vi "SelectCurDigital2DListCtrl.vi"(7 "clicked seq list?":bool, 8 "digital":dbl, 9 "digital in":refnum<vi>, 10 "column index":u16, 11 "list in":refnum<vi>) -> (3 "list out":refnum<vi>)   [LabVIEW 2018, in "Library-Ctrl.lvlib"]
uses:
  Library-Ctrl.lvlib
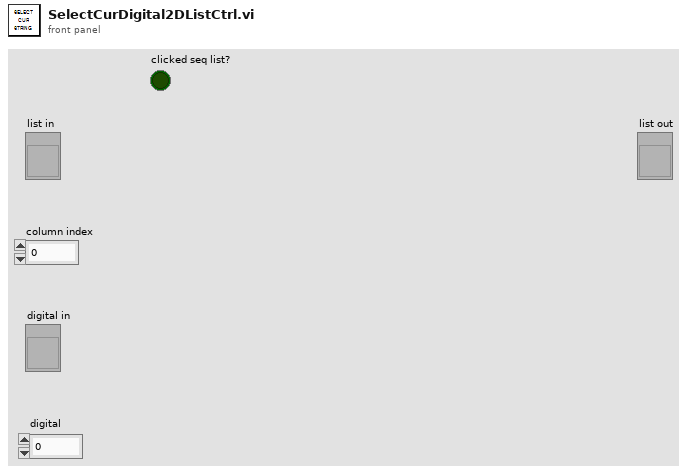
[diagram p1: front panel]
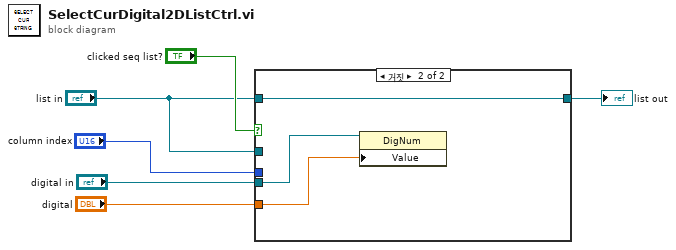
[diagram p0: block diagram]
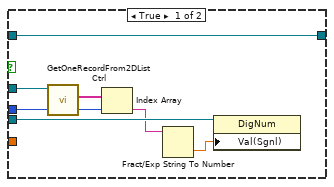
[diagram p2: hidden frame]
diagram:
  n1 = case shown="거짓" "clicked seq list?" {
    tunnel: "digital in" -> [w11 w16]
    tunnel: "digital" -> [_ w15]
    tunnel: "list in" -> [w13 _]
    tunnel: "column index" -> [w10 _]
    tunnel: [w9 w14] -> w2
    tunnel: "list in" -> [w9 w14]
    frame True {
      n2 = call "GetOneRecordFrom2DListCtrl.vi"("testcaselist in"=w13) -> ("one record"=w12:string[])  [unwired: 9 in, 1 out]
      n3 = Index Array(array=w12, index=w10) -> (element=w8:string)
      n4 = Fract/Exp String To Number(string=w8) -> (number=w7:dbl)  [unwired: 3 in, 1 out]
      n5 = property class="DigNum"(reference=w11, "Val(Sgnl)"=w7) -> ()  [unwired: 1 in, 2 out]
    }
    frame False {
      n6 = property class="DigNum"(reference=w16, "Value"=w15) -> ()  [unwired: 1 in, 2 out]
    }
  }
  "list out" <- w2
